vi "LVClass_Camera get state.vi"(0 "Camera in":refnum<class "Camera.lvclass">, 11 "error in (no error)":errorcluster) -> (4 "Camera out":refnum<class "Camera.lvclass">, 6 "is_connected?":bool, 8 "Is running?":bool, 13 "acquisition_mode":enum16{"last_image", "new_image"}(ring), 14 "synchronisation_mode":enum16{"synchronous", "asynchronous"}(ring), 15 "error out":errorcluster)   [LabVIEW 2020, in "Camera.lvclass"]
doc: "Get camera state : connected or not, running or not, acquisition mode,\nsynchronisation mode.\n\n<B>cameraIn</B> : Camera object.\n<B>cameraOut</B> : Camera object.\n<B>is_connected</B> : true if camera has been connected.\n<B>is_running</B> : true if camera has been started.\n<B>acquisition_mode</B> : image acquisition mode.\n<B>synchronization_mode</B> : image synchronization mode."
uses:
  Camera.lvclass
  Camera.lvclass/Camera.ctl
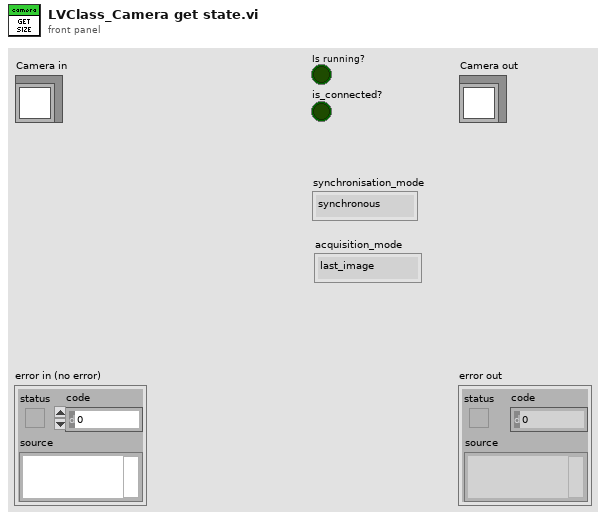
[diagram p1: front panel]
types:
  T1 = typedef "ClassID.ctl" = i64
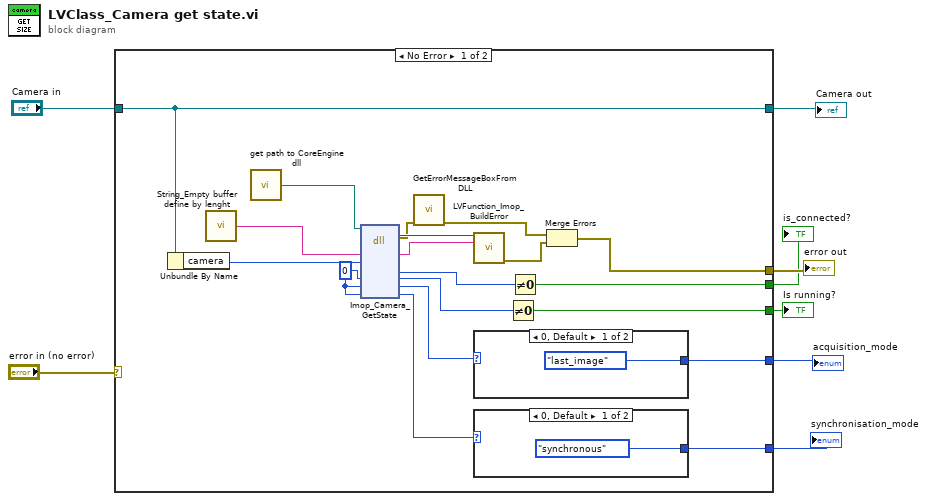
[diagram p0: block diagram]
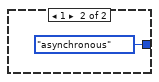
[diagram p2: hidden frame]
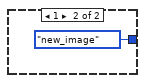
[diagram p3: hidden frame]
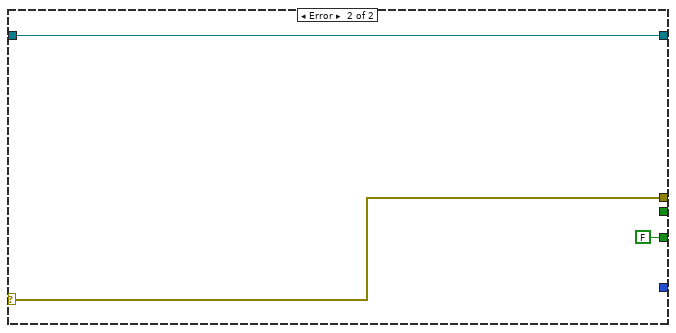
[diagram p4: hidden frame]
diagram:
  n1 = case shown="No Error" "error in (no error)" {
    selector: "error in (no error)" -> [_ w34]
    tunnel: [w19 w34] -> w5
    tunnel: [w18 w33] -> w6
    tunnel: "Camera in" -> [w18 w33]
    tunnel: [w13 FALSE] -> w4
    tunnel: [w12 _] -> w3
    tunnel: [w11 _] -> w2
    tunnel: [w9 _] -> w1
    frame No Error {
      w15 = u8 0 ("is_running")
      n2 = Unbundle By Name(w18) -> ("camera"=w24:T1)
      n3 = call "String_Empty buffer define by lenght.vi"() -> ("Empty buffer"=w27:string)  [unwired: 1 in]
      n4 = call "get path to CoreEngine dll.vi"() -> ("path to wavekit library"=w23:path)  [unwired: 14 in, 1 out]
      n5 = dll-call lib="D:/soft/HASO_v3/SVN_trunk/ImOpCoreEngine4_LV2011/DLLs/c_interface_vc100.dll" fn="Imop_Camera_GetState"(path in=w23, "message"=w27, "Camera"=w24, "is_running"=w15, "acquisition_mode"=w15, "synchronization_mode"=w15) -> (error out=w22:errorcluster, "return type"=w26:i32, "message"=w25:string, "is_connected"=w10:u8, "is_running"=w14:u8, "acquisition_mode"=w17:u8, "synchronization_mode"=w16:u8)  [unwired: 4 in, 1 out]
      n6 = call "GetErrorMessageBoxFromDLL.vi"("error IN"=w22) -> ("error OUT"=w21:errorcluster)  [unwired: 10 in]
      n7 = call "LVFunction_Imop_BuildError.vi"("code"=w26, "String to Prepend to source (\"\")"=w25) -> ("error out"=w20:errorcluster)  [unwired: 13 in]
      n8 = case shown="0, Default" w17 {
        tunnel: [enum16{"last_image", "new_image"}."last_image" ("acquisition_mode") enum16{"last_image", "new_image"}."new_image" ("acquisition_mode")] -> w11
        frame 0, Default {
        }
        frame 1 {
        }
      }
      n9 = case shown="0, Default" w16 {
        tunnel: [enum16{"synchronous", "asynchronous"}."synchronous" ("synchronisation_mode") enum16{"synchronous", "asynchronous"}."asynchronous" ("synchronisation_mode")] -> w12
        frame 0, Default {
        }
        frame 1 {
        }
      }
      n10 = Not Equal To 0?(x=w14) -> (x != 0?=w13:bool)
      n11 = Not Equal To 0?(x=w10) -> (x != 0?=w9:bool)
      n12 = Merge Errors(w21, w20) -> (w19:errorcluster)
    }
    frame Error {
    }
  }
  "error out" <- w5
  "Camera out" <- w6
  "synchronisation_mode" <- w3
  "acquisition_mode" <- w2
  "Is running?" <- w4
  "is_connected?" <- w1
